vi "CDMA_Tx_Main.vi"() -> ()   [LabVIEW 2015]
uses:
  LabviewSubVI/RFConfig/StudentMsg.ctl
  LabviewSubVI/RFConfig/RF_Config.ctl
  <vilib>/measure/maspectr.llb/FFT Spectrum (Mag-Phase) for 1 Chan (CDB).vi
  <vilib>/measure/NI_MAPro.lvlib
panel:
  out "信道1扩频前频谱":cluster{"f0":dbl, "df":dbl, "magnitude":dbl[]}(graph)
  in  "信道类型":enum16{"仿真系统", "真实系统"}(ring)
  in  "XSRP IP":string="192.168.1.145"
  in  "PC IP":string="192.168.1.215"
  out "信道1扩频后频谱":cluster{"f0":dbl, "df":dbl, "magnitude":dbl[]}(graph)
  in  "数据信道2发送字符信息":string="china,nihao"
  in  "数据信道1发送字符信息":string="helloworld"
  in  "主扰码号":u16=2 min=1 max=8
  in  "扰码组号":u16=1 min=1 max=64
  in  "信道2扩频码号":u16(ring)=2 items=["1"=1, "2"=2, "3"=3, "4"=4]
  in  "信道1扩频码号":u16(ring)=1 items=["1"=1, "2"=2, "3"=3, "4"=4]
  in  "信道2扩频因子":u16(ring)=128 items=["4"=4, "8"=8, "16"=16, "32"=32, "64"=64, "128"=128, "256"=256, "512"=512]
  in  "信道2编码方式":u16(ring)=1 items=["不编码", "1/2卷积码", "1/3卷积码"]
  in  "信道2CRC 位数":u16(ring)=8 items=["0"=0, "8"=8, "12"=12, "16"=16, "24"=24]
  in  "信道1CRC 位数":u16(ring)=8 items=["0"=0, "8"=8, "12"=12, "16"=16, "24"=24]
  in  "?":T1={"发射频率"=2000000000, "发射衰减"=20, "接收频率"=2000000000, "接收增益"=0, "接收通道"=enum."RxCh1", "发射通道"=enum."TxCh1"} {"接收增益" max=40 format="%.0fdB"; "接收频率" min=70000000 max=6000000000 format="%.9pHz"; "发射衰减" max=90 format="%.0fdB"; "发射频率" min=70000000 max=6000000000 format="%.9pHz"}
  in  "信道1扩频因子":u16(ring)=128 items=["4"=4, "8"=8, "16"=16, "32"=32, "64"=64, "128"=128]
  in  "信道1编码方式":u16(ring)=1 items=["不编码", "1/2卷积码", "1/3卷积码"]
  out "实验学生信息":T2={"姓名"="XXX\n", "学号"="XXX", "班级"="XXX", "学校"="XXX"}
  # "基于XSRP软件无线电平台的CDMA通信系统发射机设计"
  # "实验参数设置"
  # "实验学生信息"
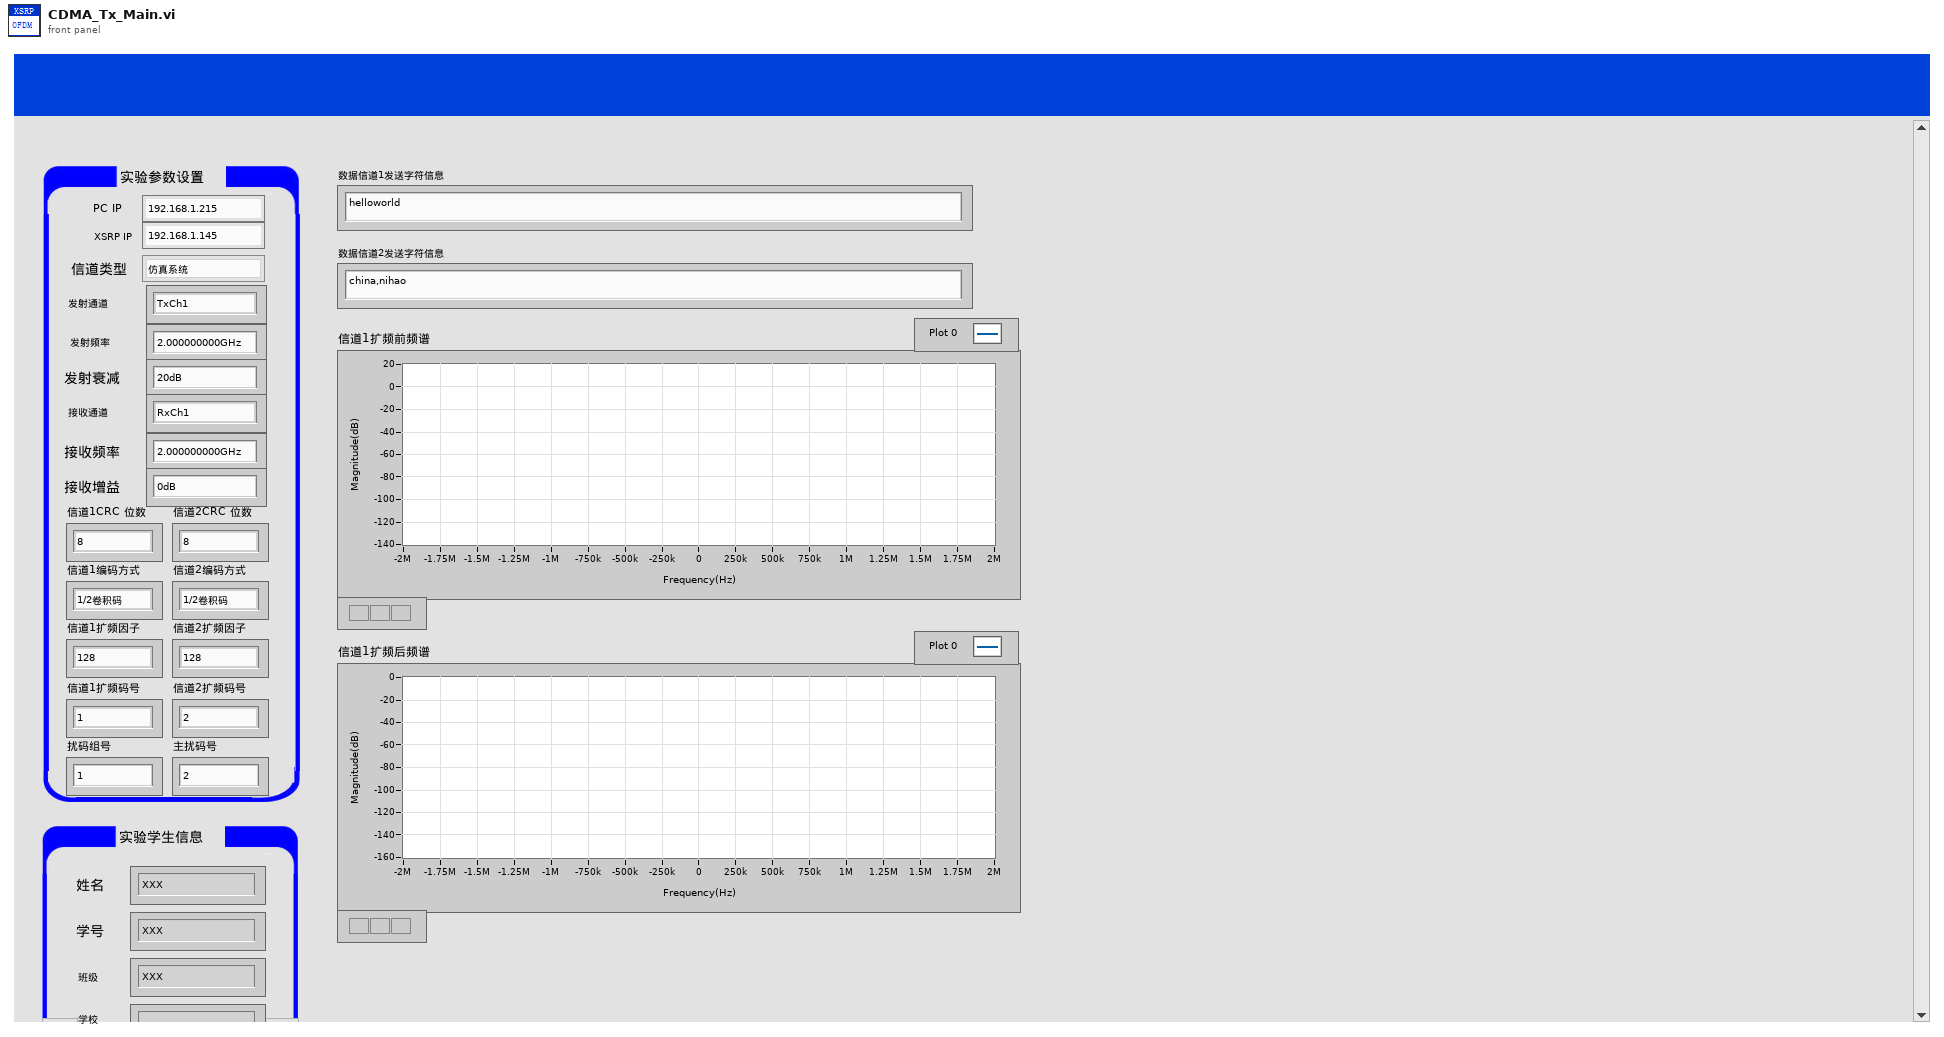
[diagram p1: front panel]
types:
  T1 = typedef "RF_Config.ctl" = cluster{"发射频率":u64, "发射衰减":u8, "接收频率":u64, "接收增益":u8, "接收通道":enum16{"RxCh1", "RxCh2"}, "发射通道":enum16{"TxCh1", "TxCh2"}}
  T2 = typedef "StudentMsg.ctl" = cluster{"姓名":string, "学号":string, "班级":string, "学校":string}
  T3 = cluster{"dB On (F)":bool, "unwrap phase (F)":bool, "convert to degree (F)":bool}
  T4 = cluster{"接收通道":enum16{"RxCh1", "RxCh2"}, "接收频率":u32, "接收增益":u8}
  T5 = cluster{"发射通道":enum16{"TxCh1", "TxCh2"}, "发射频率":u32, "发射衰减":u8}
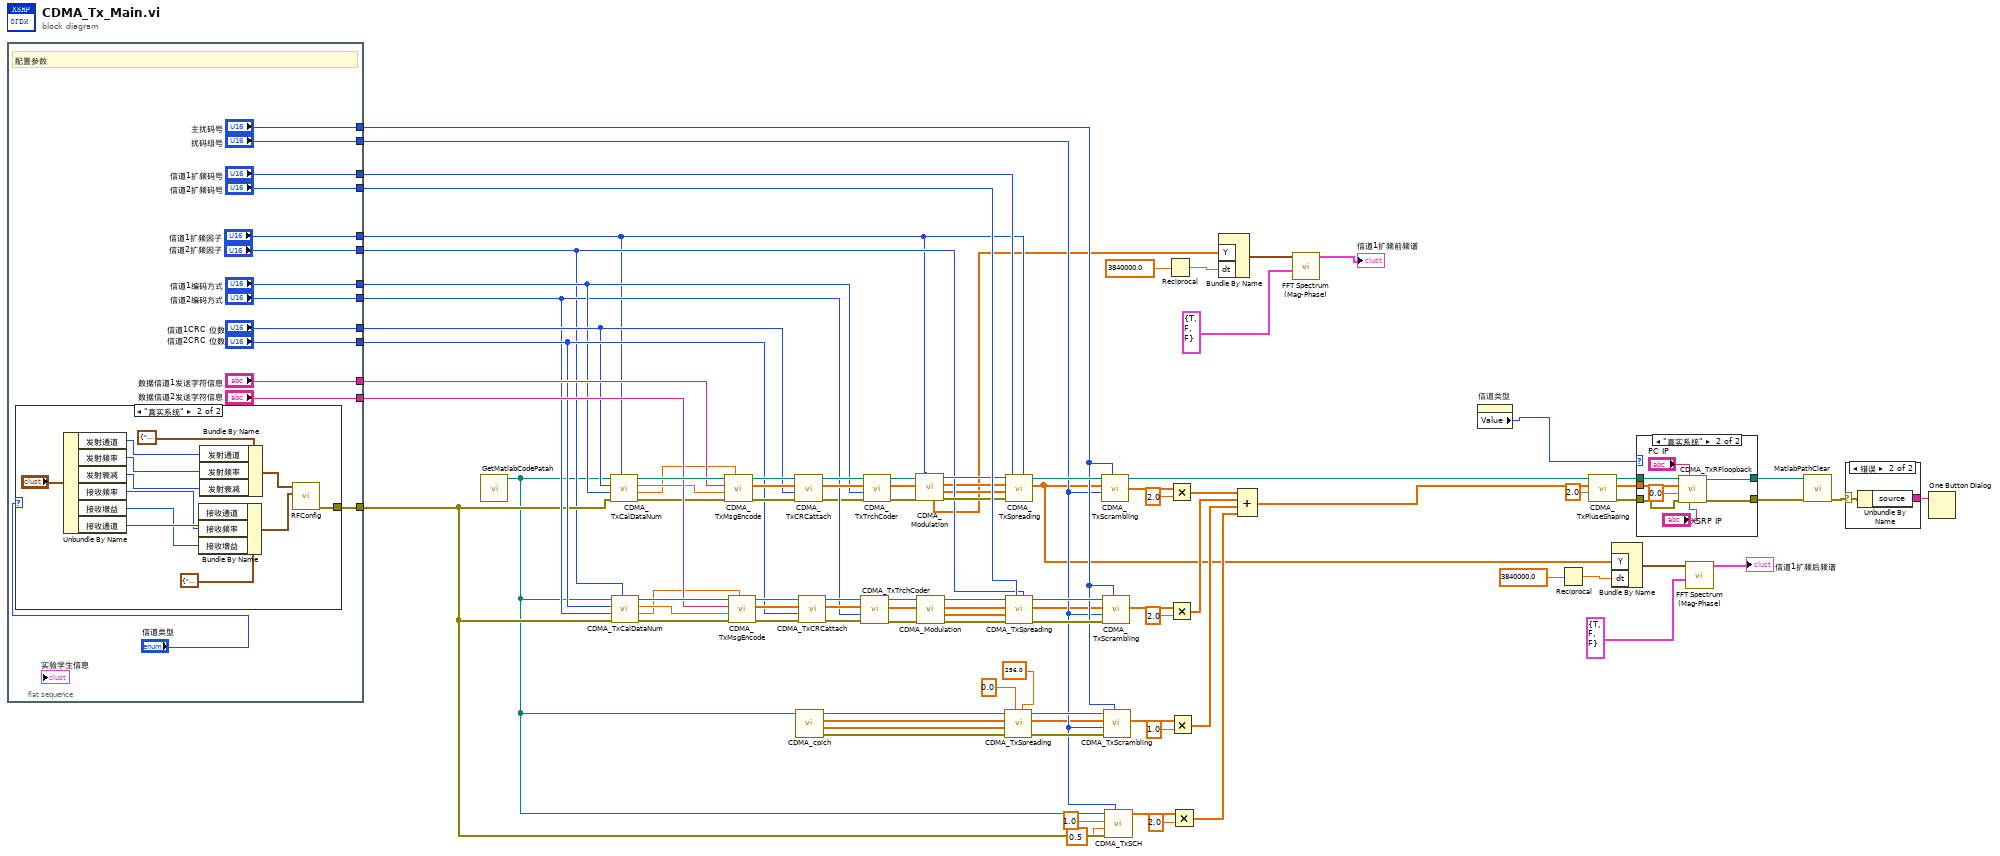
[diagram p0: block diagram]
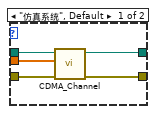
[diagram p2: hidden frame]
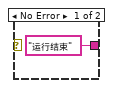
[diagram p3: hidden frame]
diagram:
  n1 = flat-sequence {
    tunnel: ["信道1编码方式"] -> w66
    tunnel: ["信道1扩频因子"] -> w6
    tunnel: [w110] -> w56
    tunnel: ["信道1CRC 位数"] -> w71
    tunnel: ["信道2CRC 位数"] -> w72
    tunnel: ["信道2编码方式"] -> w65
    tunnel: ["信道2扩频因子"] -> w26
    tunnel: ["数据信道1发送字符信息"] -> w86
    tunnel: ["数据信道2发送字符信息"] -> w84
    tunnel: ["信道1扩频码号"] -> w27
    tunnel: ["信道2扩频码号"] -> w63
    tunnel: ["扰码组号"] -> w55
    tunnel: ["主扰码号"] -> w57
    frame #0 {
      # "配置参数"
      n2 = case shown="\"真实系统\"" "信道类型" {
        tunnel: [_ w113] -> w110
        frame "仿真系统" {
        }
        frame "真实系统" {
          n3 = Unbundle By Name("?") -> ("发射通道"=w121:enum16{"TxCh1", "TxCh2"}, "发射频率"=w120:u64, "发射衰减"=w119:u8, "接收频率"=w115:u64, "接收增益"=w116:u8, "接收通道"=w117:enum16{"RxCh1", "RxCh2"})
          n4 = Bundle By Name(cluster=T4 {"接收通道"=enum."RxCh1", "接收频率"=0, "接收增益"=0} ("接收参数设置"), "接收通道"=w117, "接收频率"=w115, "接收增益"=w116) -> (w114:T4)
          n5 = Bundle By Name(cluster=T5 {"发射通道"=enum."TxCh1", "发射频率"=0, "发射衰减"=0} ("发射参数设置"), "发射通道"=w121, "发射频率"=w120, "发射衰减"=w119) -> (w123:T5)
          n6 = call "RFConfig.vi"("接收参数设置"=w114, "发射参数设置"=w123) -> ("error out"=w113:errorcluster)  [unwired: 9 in]
        }
      }
    }
  }
  n7 = call "GetMatlabCodePatah.vi"() -> ("MatlabCodePath"=w12:path)  [unwired: 11 in]
  n8 = call "CDMA_TxCalDataNum.vi"("ch_sf_tx"=w6, "error in (no error)"=w56, "coder_type"=w66, "crc_num"=w71, "Path"=w12) -> ("error out"=w78:errorcluster, "ch_cap"=w80:dbl, "ch_bit_len"=w83:dbl, "Path Out"=w93:path)  [unwired: 3 in]
  n9 = call "CDMA_TxCalDataNum.vi"("ch_sf_tx"=w26, "error in (no error)"=w56, "coder_type"=w65, "crc_num"=w72, "Path"=w12) -> ("error out"=w79:errorcluster, "ch_cap"=w81:dbl, "ch_bit_len"=w82:dbl, "Path Out"=w85:path)  [unwired: 3 in]
  n10 = call "CDMA_TxMsgEncode.vi"("ch_cap"=w80, "error in (no error)"=w78, "ch_bit_len"=w83, "ch_char_msg"=w86, "Path"=w93) -> ("error out"=w77:errorcluster, "pdch_data"=w76:dbl[], "Path Out"=w92:path)  [unwired: 4 in]
  n11 = call "CDMA_TxMsgEncode.vi"("ch_cap"=w81, "error in (no error)"=w79, "ch_bit_len"=w82, "ch_char_msg"=w84, "Path"=w85) -> ("error out"=w73:errorcluster, "pdch_data"=w75:dbl[], "Path Out"=w74:path)  [unwired: 4 in]
  n12 = call "CDMA_TxCRCattach.vi"("error in (no error)"=w77, "crc_num"=w71, "pdch_data"=w76, "Path"=w92) -> ("error out"=w64:errorcluster, "attach_crc_data"=w70:dbl[], "Path Out"=w91:path)  [unwired: 5 in]
  n13 = call "CDMA_cpich.vi"("Path"=w12) -> ("error out"=w10:errorcluster, "data_q"=w13:cdb[], "data_i"=w14:cdb[], "Path Out"=w11:path)  [unwired: 7 in]
  n14 = call "CDMA_TxCRCattach.vi"("error in (no error)"=w73, "crc_num"=w72, "pdch_data"=w75, "Path"=w74) -> ("error out"=w67:errorcluster, "attach_crc_data"=w68:dbl[], "Path Out"=w69:path)  [unwired: 5 in]
  n15 = call "CDMA_TxTrchCoder.vi"("error in (no error)"=w67, "coder_type"=w65, "attach_crc_data"=w68, "Path"=w69) -> ("error out"=w19:errorcluster, "tch_code_data"=w20:dbl[], "Path Out"=w22:path)  [unwired: 5 in]
  n16 = call "CDMA_TxTrchCoder.vi"("error in (no error)"=w64, "coder_type"=w66, "attach_crc_data"=w70, "Path"=w91) -> ("error out"=w30:errorcluster, "tch_code_data"=w31:dbl[], "Path Out"=w32:path)  [unwired: 5 in]
  n17 = call "CDMA_Modulation.vi"("ch1_sf_tx"=w6, "error in (no error)"=w30, "sf_data"=w31, "Path"=w32) -> ("error out"=w28:errorcluster, "data_q"=w23:dbl[], "data_i"=w24:dbl[], "Path Out"=w29:path, "output_data"=w2:cdb[])  [unwired: 3 in]
  n18 = call "CDMA_Modulation.vi"("error in (no error)"=w19, "sf_data"=w20, "Path"=w22) -> ("error out"=w16:errorcluster, "data_q"=w17:dbl[], "data_i"=w18:dbl[], "Path Out"=w21:path)  [unwired: 4 in, 1 out]
  n19 = call "CDMA_TxSpreading.vi"("ch_sf_tx"=256.0, "ch_code_tx"=0.0, "error in (no error)"=w10, "input_dataq"=w13, "input_datai"=w14, "Path"=w11) -> ("error out"=w58:errorcluster, "sf_data"=w33:cdb[], "Path Out"=w59:path)  [unwired: 3 in]
  n20 = call "CDMA_TxSpreading.vi"("ch_sf_tx"=w6, "ch_code_tx"=w27, "error in (no error)"=w28, "input_dataq"=w23, "input_datai"=w24, "Path"=w29) -> ("sf_data"=w35:cdb[], "Path Out"=w90:path)  [unwired: 3 in, 1 out]
  n21 = call "CDMA_TxSpreading.vi"("ch_sf_tx"=w26, "ch_code_tx"=w63, "error in (no error)"=w16, "input_dataq"=w17, "input_datai"=w18, "Path"=w21) -> ("error out"=w61:errorcluster, "sf_data"=w34:cdb[], "Path Out"=w62:path)  [unwired: 3 in]
  n22 = call "CDMA_TxScrambling.vi"("scramble_num_tx"=w57, "sc_group_num_tx"=w55, "sf_data"=w35, "Path"=w90) -> ("sc_data"=w39:cdb[], "Path Out"=w41:path)  [unwired: 5 in, 1 out]
  n23 = call "CDMA_TxScrambling.vi"("scramble_num_tx"=w57, "error in (no error)"=w61, "sc_group_num_tx"=w55, "sf_data"=w34, "Path"=w62) -> ("sc_data"=w50:cdb[])  [unwired: 4 in, 2 out]
  n24 = call "CDMA_TxScrambling.vi"("scramble_num_tx"=w57, "error in (no error)"=w58, "sc_group_num_tx"=w55, "sf_data"=w33, "Path"=w59) -> ("sc_data"=w48:cdb[])  [unwired: 4 in, 2 out]
  n25 = call "CDMA_TxSCH.vi"("sc_group_num_tx"=w55, "error in (no error)"=w56, "Gs"=0.5, "Gp"=1.0, "Path"=w12) -> ("sch_data"=w46:cdb[])  [unwired: 5 in, 1 out]
  n26 = Reciprocal(x=3840000.0) -> (1/x=w8:dbl)
  n27 = Multiply(x=w39, y=2.0) -> (x*y=w45:cdb[])
  n28 = Multiply(x=w50, y=2.0) -> (x*y=w44:cdb[])
  n29 = Multiply(x=w48, y=1.0) -> (x*y=w43:cdb[])
  n30 = Multiply(x=w46, y=2.0) -> (x*y=w42:cdb[])
  n31 = Bundle By Name("Y"=w2, "dt"=w8) -> (w7:waveform(cdb))  [unwired: 1 in]
  n32 = Compound Arithmetic op=ADD(w45, w44, w43, w42) -> (w5:cdb[])
  n33 = call-poly <vilib>:"FFT Spectrum (Mag-Phase).vi"("view"=T3 {"dB On (F)"=TRUE, "unwrap phase (F)"=FALSE, "convert to degree (F)"=FALSE}, "time signal"=w7) -> ("magnitude"=→"信道1扩频前频谱":cluster{"f0":dbl, "df":dbl, "magnitude":dbl[]})  [unwired: 5 in, 4 out]
  n34 = property on="信道类型" class="Enum (严格)"() -> ("Value"=w15:enum16{"仿真系统", "真实系统"})  [unwired: 2 in, 2 out]
  n35 = Reciprocal(x=3840000.0) -> (1/x=w97:dbl)
  n36 = call "CDMA_TxPluseShaping.vi"("sampleRate"=2.0, "sc_data"=w5, "Path"=w41) -> ("error out"=w38:errorcluster, "tx_data"=w37:cdb[], "Path Out"=w87:path)  [unwired: 6 in]
  n37 = Bundle By Name("Y"=w35, "dt"=w97) -> (w36:waveform(cdb))  [unwired: 1 in]
  n38 = case shown="\"真实系统\"" w15 {
    tunnel: [w129 w132] -> w89
    tunnel: [w128 w133] -> w88
    tunnel: w87 -> [w127 w137]
    tunnel: w38 -> [w126 w134]
    tunnel: w37 -> [w125 w136]
    frame "仿真系统", Default {
      n39 = call "CDMA_Channel.vi"("error in (no error)"=w126, "tx_data"=w125, "Path"=w127) -> ("error out"=w128:errorcluster, "Path Out"=w129:path)  [unwired: 6 in, 1 out]
    }
    frame "真实系统" {
      n40 = call "CDMA_TxRFloopback.vi"("xsrpip"="XSRP IP", "pcip"="PC IP", "error in (no error)"=w134, "system_type"=0.0, "tx_data"=w136, "Path In"=w137) -> ("error out"=w133:errorcluster, "Path Out"=w132:path)  [unwired: 4 in]
    }
  }
  n41 = call-poly <vilib>:"FFT Spectrum (Mag-Phase).vi"("view"=T3 {"dB On (F)"=TRUE, "unwrap phase (F)"=FALSE, "convert to degree (F)"=FALSE}, "time signal"=w36) -> ("magnitude"=→"信道1扩频后频谱":cluster{"f0":dbl, "df":dbl, "magnitude":dbl[]})  [unwired: 5 in, 4 out]
  n42 = call "MatlabPathClear.vi"("error in"=w88, "Path"=w89) -> ("error out"=w94:errorcluster)  [unwired: 9 in]
  n43 = case shown="错误" w94 {
    selector: w94 -> [_ w139]
    tunnel: ["运行结束" ("source") w140] -> w95
    frame No Error {
    }
    frame Error {
      n44 = Unbundle By Name(w139) -> ("source"=w140:string)
    }
  }
  n45 = One Button Dialog(message=w95) -> ()  [unwired: 1 in, 1 out]
